vi "parseValue.vi"(8 "error in (no error)":errorcluster, 10 "message":string, 11 "SpectrographClientCommunicator in":refnum<class "SpectrographClientCommunicator.lvclass">) -> (0 "error out":errorcluster, 2 "Output":string, 3 "SpectrographClientCommunicator out":refnum<class "SpectrographClientCommunicator.lvclass">)   [LabVIEW 2016, in "SpectrographClientCommunicator.lvclass"]
uses:
  SpectrographClientCommunicator.lvclass
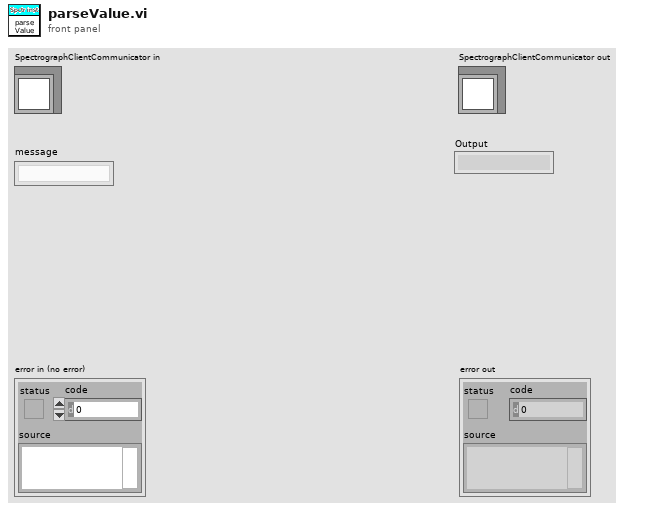
[diagram p1: front panel]
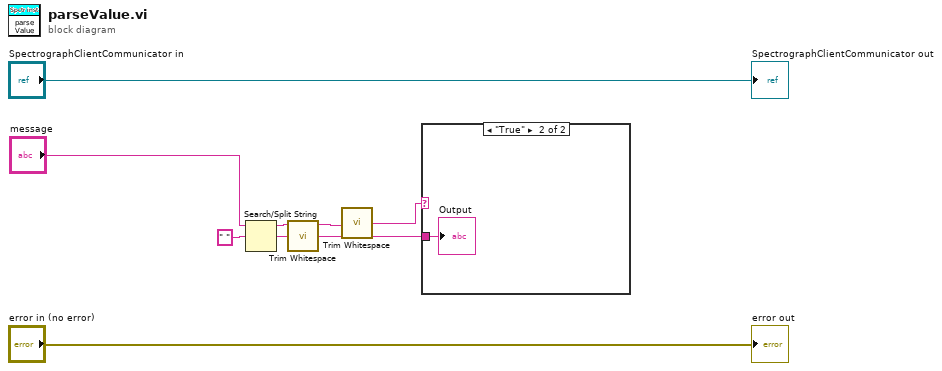
[diagram p0: block diagram]
diagram:
  n1 = Search/Split String(string="message", search string/char (-)=" ") -> (substring before match=w4:string, match + rest of string=w5:string)  [unwired: 1 in, 1 out]
  n2 = call <vilib>:"Trim Whitespace.vi"("string"=w5) -> ("trimmed string"=w1:string)  [unwired: 1 in]
  n3 = call <vilib>:"Trim Whitespace.vi"("string"=w4) -> ("trimmed string"=w2:string)  [unwired: 1 in]
  n4 = case shown="\"True\"" w2 {
    tunnel: w1 -> [_ w9]
    frame "False", Default {
    }
    frame "True" {
      "Output" <- w9
    }
  }
  "error out" <- "error in (no error)"
  "SpectrographClientCommunicator out" <- "SpectrographClientCommunicator in"
